vi "求三角形面积.vi"() -> ()   [LabVIEW 2018]
panel:
  out "S":dbl
  in  "C":dbl
  in  "B":dbl
  in  "A":dbl
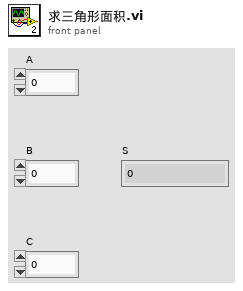
[diagram p1: front panel]
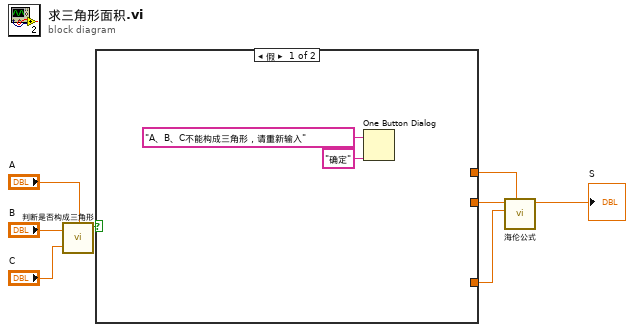
[diagram p0: block diagram]
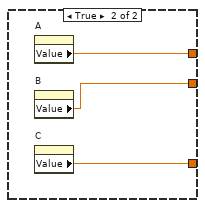
[diagram p2: hidden frame]
diagram:
  n1 = call "判断是否构成三角形.vi"("B"="B", "C"="C", "A"="A") -> ("A、B、C是否构成三角形"=w5:bool)  [unwired: 6 in]
  n2 = case shown="假" w5 {
    tunnel: [_ w13] -> w4
    tunnel: [_ w12] -> w3
    tunnel: [_ w11] -> w2
    frame False {
      n3 = One Button Dialog(message="A、B、C不能构成三角形，请重新输入" ("消息"), button name ("OK")="确定" ("按钮名称（“确定”）")) -> ()  [unwired: 1 out]
    }
    frame True {
      n4 = property on="A" class="DigNum (严格)"() -> ("Value"=w13:dbl)  [unwired: 2 in, 2 out]
      n5 = property on="B" class="DigNum (严格)"() -> ("Value"=w12:dbl)  [unwired: 2 in, 2 out]
      n6 = property on="C" class="DigNum (严格)"() -> ("Value"=w11:dbl)  [unwired: 2 in, 2 out]
    }
  }
  n7 = call "海伦公式.vi"("A"=w4, "C"=w2, "B"=w3) -> ("S"=→"S":dbl)  [unwired: 8 in]
